vi "board_stepcompare.vi"(0 "Aggregate Shapes":T4(array[cluster]), 1 "Dimensions":T5, 2 "Board Layout":cluster{"Piece Type":T2, "Team Color":T3}[][](array[cluster])) -> (7 "Changelist":T1[](array[typedef]))   [LabVIEW 2015]
uses:
  chess_piecetype_enum.ctl
  chess_teamcolor_enum.ctl
  chess_poschangeinfo_cluster.ctl
panel:
  in  "cluster def":T1
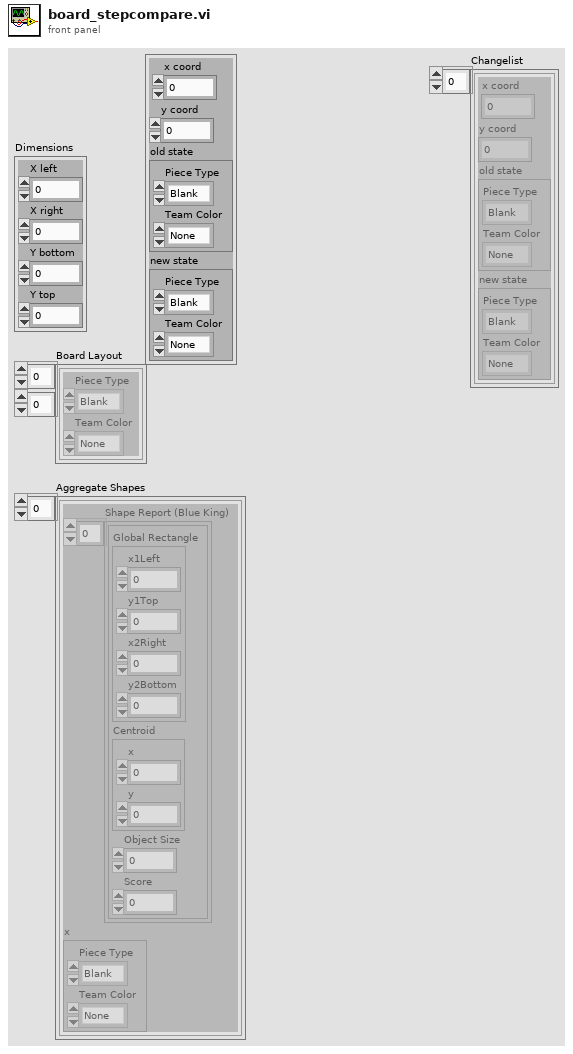
[diagram p1: front panel]
types:
  T1 = typedef "chess_poschangeinfo_cluster.ctl" = cluster{"x coord":i32, "y coord":i32, "old state":cluster{"Piece Type":T2, "Team Color":T3}, "new state":cluster{"Piece Type":T2, "Team Color":T3}}
  T2 = typedef "chess_piecetype_enum.ctl" = enum16{"Blank", "Pawn", "Rook", "Knight", "Bishop", "Queen", "King"}
  T3 = typedef "chess_teamcolor_enum.ctl" = enum16{"None", "Red", "Blue"}
  T4 = cluster{"Shape Report (Blue King)":cluster{"Global Rectangle":cluster{"x1Left":i32, "y1Top":i32, "x2Right":i32, "y2Bottom":i32}, "Centroid":cluster{"x":sgl, "y":sgl}, "Object Size":u32, "Score":dbl}[], "x":cluster{"Piece Type":T2, "Team Color":T3}}[]
  T5 = cluster{"X left":dbl, "X right":dbl, "Y bottom":dbl, "Y top":dbl}
  T6 = cluster{"Global Rectangle":cluster{"x1Left":i32, "y1Top":i32, "x2Right":i32, "y2Bottom":i32}, "Centroid":cluster{"x":sgl, "y":sgl}, "Object Size":u32, "Score":dbl}[]
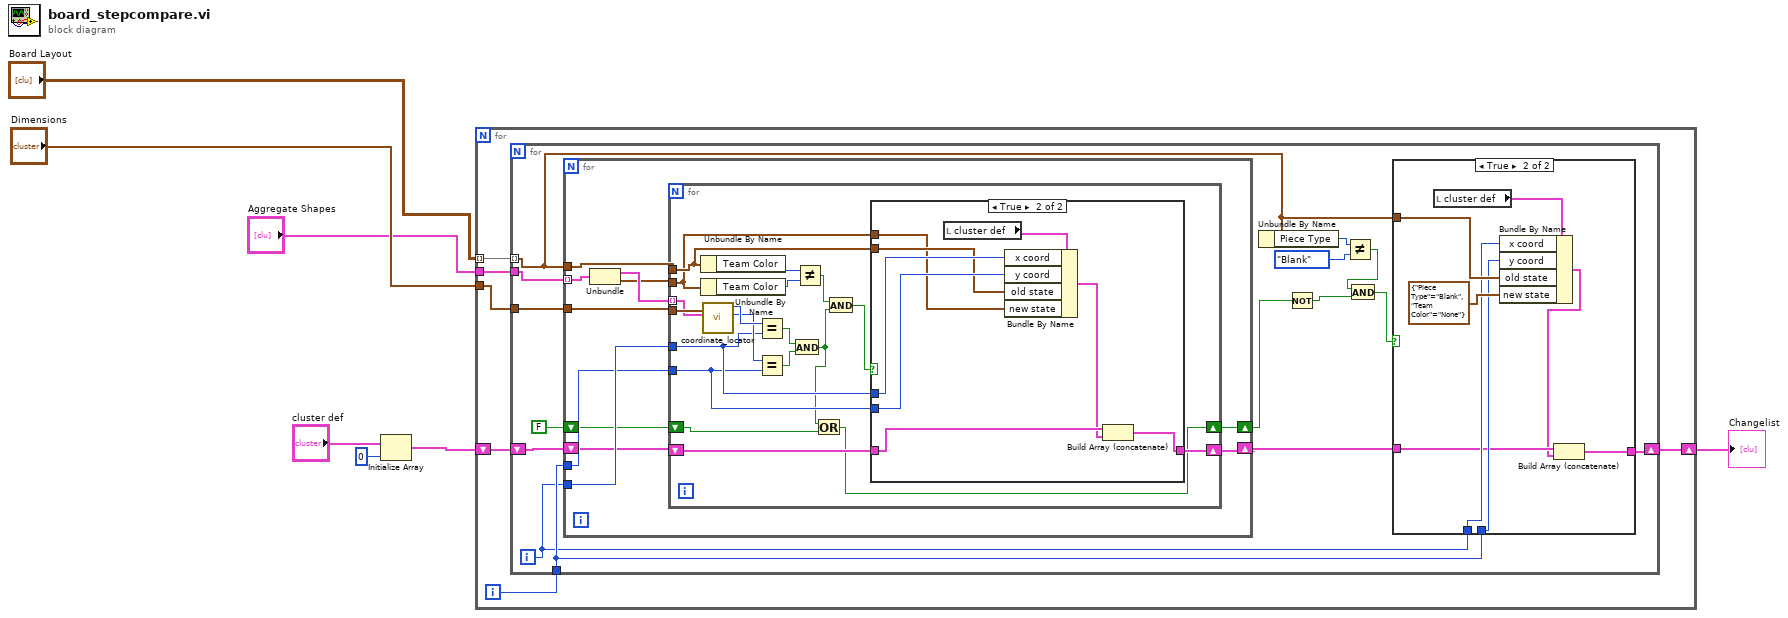
[diagram p0: block diagram]
diagram:
  n1 = Initialize Array("cluster def", 0 ("dimension size")) -> (w3:T1[])
  n2 = for {
    tunnel: "Board Layout" -> [w13] mode=indexing
    tunnel: "Aggregate Shapes" -> [w12]
    tunnel: "Dimensions" -> [w10]
    shift-right: [w8] -> w2
    shift-left: w3 -> [w9]
    i -> [w11]
    n3 = for {
      tunnel: w13 -> [w18] mode=indexing
      tunnel: w12 -> [w26]
      tunnel: w11 -> [w17]
      tunnel: w10 -> [w28]
      shift-right: [w14] -> w8
      shift-left: w9 -> [w27]
      i -> [w16]
      n4 = for {
        tunnel: w26 -> [w48] mode=indexing
        tunnel: w18 -> [w46]
        tunnel: w17 -> [w43]
        tunnel: w16 -> [w44]
        tunnel: w28 -> [w40]
        shift-right: [w41] -> w15
        shift-left: w27 -> [w42]
        shift-right: [w38] -> w21
        shift-left: FALSE -> [w39]
        n5 = Unbundle(w48) -> ("Shape Report (Blue King)"=w47:T6, "x"=w45:cluster{"Piece Type":T2, "Team Color":T3})
        n6 = for {
          tunnel: w47 -> [w66] mode=indexing
          tunnel: w46 -> [w53]
          tunnel: w40 -> [w67]
          tunnel: w45 -> [w52]
          tunnel: w44 -> [w55]
          tunnel: w43 -> [w54]
          shift-right: [w56] -> w41
          shift-left: w42 -> [w57]
          shift-right: [w49] -> w38
          shift-left: w39 -> [w50]
          n7 = Unbundle By Name(w53) -> ("Team Color"=w63:T3)
          n8 = Unbundle By Name(w52) -> ("Team Color"=w62:T3)
          n9 = call "coordinate_locator.vi"("Shape Cluster"=w66, "Dimensions"=w67) -> ("y coord"=w64:i32, "x coord"=w65:i32)  [unwired: 8 in]
          n10 = Equal?(x=w65, y=w55) -> (x = y?=w61:bool)
          n11 = Equal?(x=w64, y=w54) -> (x = y?=w60:bool)
          n12 = And(x=w61, y=w60) -> (x .and. y?=w51:bool)
          n13 = Not Equal?(x=w63, y=w62) -> (x != y?=w59:bool)
          n14 = Or(x=w51, y=w50) -> (x .or. y?=w49:bool)
          n15 = And(x=w59, y=w51) -> (x .and. y?=w58:bool)
          n16 = case shown="True" w58 {
            tunnel: w57 -> [w68 w72]
            tunnel: [w68 w71] -> w56
            tunnel: w55 -> [_ w76]
            tunnel: w54 -> [_ w75]
            tunnel: w53 -> [_ w74]
            tunnel: w52 -> [_ w73]
            frame False {
            }
            frame True {
              n17 = local read "cluster def"() -> (w69:T1)
              n18 = Bundle By Name(cluster=w69, "x coord"=w76, "y coord"=w75, "old state"=w74, "new state"=w73) -> (w70:T1)
              n19 = Build Array (concatenate)(w72, w70) -> (w71:T1[])
            }
          }
        }
      }
      n20 = Unbundle By Name(w18) -> ("Piece Type"=w24:T2)
      n21 = Not(x=w21) -> (.not. x?=w20:bool)
      n22 = Not Equal?(x=w24, y=chess_piecetype_enum."Blank" ("Piece Type")) -> (x != y?=w22:bool)
      n23 = And(x=w22, y=w20) -> (x .and. y?=w19:bool)
      n24 = case shown="True" w19 {
        tunnel: w18 -> [_ w36]
        tunnel: w17 -> [_ w35]
        tunnel: w16 -> [_ w34]
        tunnel: w15 -> [w29 w33]
        tunnel: [w29 w30] -> w14
        frame False {
        }
        frame True {
          n25 = local read "cluster def"() -> (w32:T1)
          n26 = Bundle By Name(cluster=w32, "x coord"=w34, "y coord"=w35, "old state"=w36, "new state"=cluster{"Piece Type":T2, "Team Color":T3} {"Piece Type"=enum."Blank", "Team Color"=enum."None"}) -> (w31:T1)
          n27 = Build Array (concatenate)(w33, w31) -> (w30:T1[])
        }
      }
    }
  }
  "Changelist" <- w2
